vi "Parse Access Control Policy.vi"(11 "Body":string) -> (3 "Access Control Policy":T1)   [LabVIEW 2015, in "NI_AWS_S3.lvlib"]
uses:
  NI_AWS_S3.lvlib
  Access Control Policy.ctl
  User.ctl
  Grantee-Permission Pair.ctl
  Permission.ctl
  XML Parsing/NI_XML Parsing.lvlib
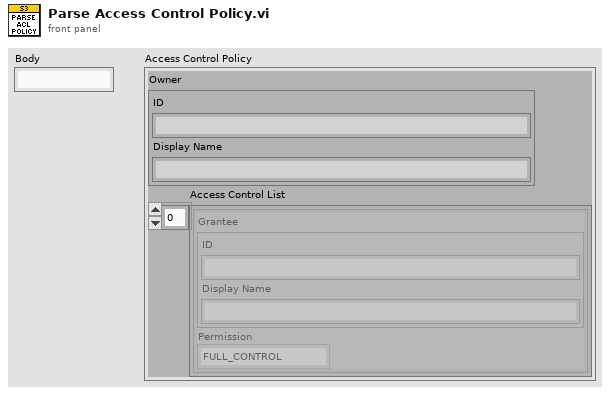
[diagram p1: front panel]
types:
  T1 = typedef "NI_AWS_S3.lvlib/Access Control Policy.ctl" = cluster{"Owner":T2, "Access Control List":T3[]}
  T2 = typedef "NI_AWS_S3.lvlib/User.ctl" = cluster{"ID":string, "Display Name":string}
  T3 = typedef "NI_AWS_S3.lvlib/Grantee-Permission Pair.ctl" = cluster{"Grantee":T2, "Permission":T4}
  T4 = typedef "NI_AWS_S3.lvlib/Permission.ctl" = enum16{"FULL_CONTROL", "WRITE", "WRITE_ACP", "READ", "READ_ACP"}
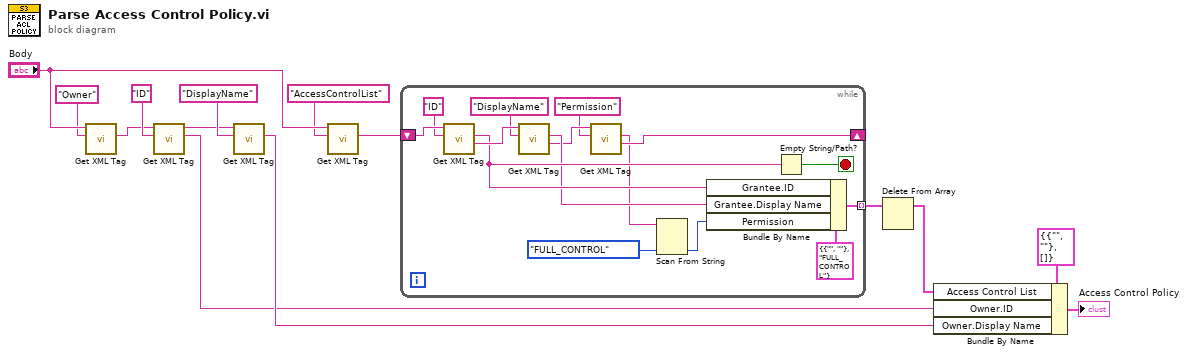
[diagram p0: block diagram]
diagram:
  n1 = call "Get XML Tag.vi"("Tag name"="Owner", "XML String in"="Body") -> ("Tag value"=w4:string)  [unwired: 5 in, 4 out]
  n2 = call "Get XML Tag.vi"("Tag name"="ID", "XML String in"=w4) -> ("Tag value"=w8:string, "XML String dup"=w5:string)  [unwired: 5 in, 3 out]
  n3 = call "Get XML Tag.vi"("Tag name"="DisplayName", "XML String in"=w5) -> ("Tag value"=w9:string)  [unwired: 5 in, 4 out]
  n4 = call "Get XML Tag.vi"("Tag name"="AccessControlList", "XML String in"="Body") -> ("Tag value"=w12:string)  [unwired: 5 in, 4 out]
  n5 = while {
    shift-right: [w20] -> _
    shift-left: w12 -> [w29]
    tunnel: [w25] -> w13 mode=indexing
    stop <- w15 stop-if-true
    n6 = call "Get XML Tag.vi"("Tag name"="ID", "XML String in"=w29) -> ("Remaining string"=w27:string, "Tag value"=w23:string)  [unwired: 5 in, 3 out]
    n7 = call "Get XML Tag.vi"("Tag name"="DisplayName", "XML String in"=w27) -> ("Remaining string"=w21:string, "Tag value"=w22:string)  [unwired: 5 in, 3 out]
    n8 = call "Get XML Tag.vi"("Tag name"="Permission", "XML String in"=w21) -> ("Remaining string"=w20:string, "Tag value"=w18:string)  [unwired: 5 in, 3 out]
    n9 = Scan From String(input string=w18, default 1=Permission."FULL_CONTROL" ("Permission")) -> (output 1=w16:T4)  [unwired: 3 in, 3 out]
    n10 = Bundle By Name(cluster=T3 {"Grantee"={"ID"="", "Display Name"=""}, "Permission"=enum."FULL_CONTROL"} ("User-Permission Pair"), "Grantee.ID"=w23, "Grantee.Display Name"=w22, "Permission"=w16) -> (w25:T3)
    n11 = Empty String/Path?(string/path=w23) -> (empty?=w15:bool)
  }
  n12 = Delete From Array(array=w13) -> (array with subset deleted=w14:T3[])  [unwired: 2 in, 1 out]
  n13 = Bundle By Name(cluster=T1 {"Owner"={"ID"="", "Display Name"=""}, "Access Control List"=[]} ("Access Control Policy"), "Access Control List"=w14, "Owner.ID"=w8, "Owner.Display Name"=w9) -> (→"Access Control Policy":T1)
